vi "subvi_calc.vi"(4 "Function":enum16{"+", "-", "/", "*", "sqrt", "%"}(ring), 8 "Input in":dbl, 9 "Input 1":dbl) -> (3 "Answer":dbl)   [LabVIEW 2020]
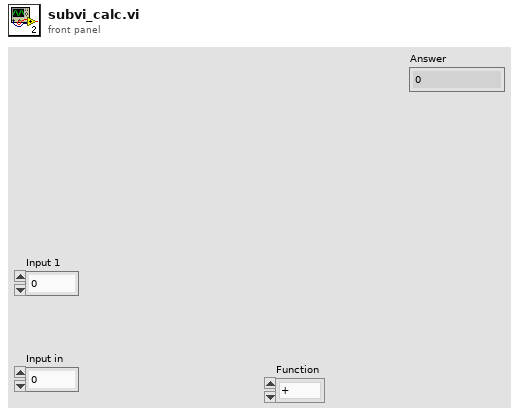
[diagram p1: front panel]
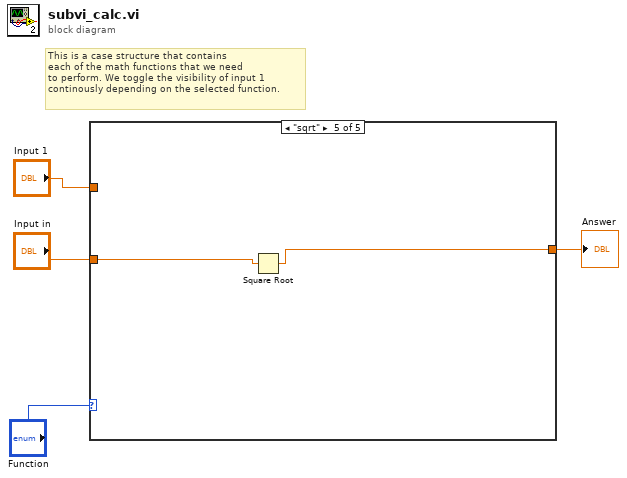
[diagram p0: block diagram]
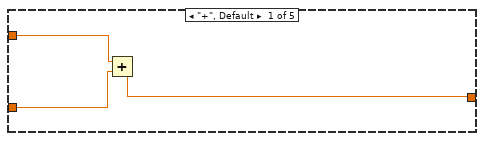
[diagram p2: hidden frame]
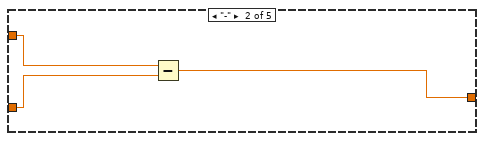
[diagram p3: hidden frame]
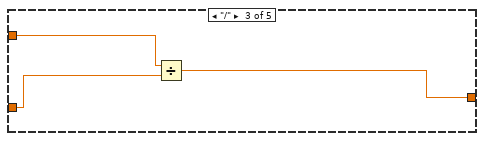
[diagram p4: hidden frame]
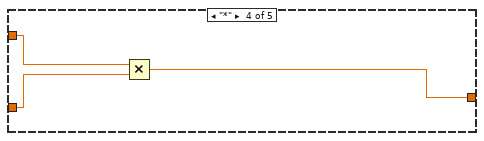
[diagram p5: hidden frame]
diagram:
  # "This is a case structure that contains\neach of the math functions that we need \nto perform. We toggle the visibility of input 1\ncontinously depending on the selected function."
  n1 = case shown="\"sqrt\"" "Function" {
    tunnel: "Input 1" -> [w7 w10 w13 w16 _]
    tunnel: "Input in" -> [w6 w9 w12 w15 w18]
    tunnel: [w5 w8 w11 w14 w17] -> w3
    frame "+", Default {
      n2 = Add(x=w7, y=w6) -> (x+y=w5:dbl)
    }
    frame "-" {
      n3 = Subtract(x=w10, y=w9) -> (x-y=w8:dbl)
    }
    frame "/" {
      n4 = Divide(x=w13, y=w12) -> (x/y=w11:dbl)
    }
    frame "*" {
      n5 = Multiply(x=w16, y=w15) -> (x*y=w14:dbl)
    }
    frame "sqrt" {
      n6 = Square Root(x=w18) -> (sqrt(x)=w17:dbl)
    }
  }
  "Answer" <- w3
